vi "write memory.vi"(8 "error in (no error)":errorcluster, 10 "IQ data":u64[](array[numeric]), 11 "USRP_1_x_200MHz in":refnum<class "USRP_1_x_200MHz.lvclass">) -> (0 "error out":errorcluster, 3 "USRP_1_x_200MHz out":refnum<class "USRP_1_x_200MHz.lvclass">)   [LabVIEW 2021, in "USRP_1_x_200MHz.lvclass"]
uses:
  USRP_1_x_200MHz.lvclass
  USRP_1_x_200MHz.lvclass/USRP_1_x_200MHz.ctl
  <vilib>/rvi/interface/nirviMethod/nirviMethod.xnode
  <vilib>/FPGAPlugInAG/Dynamic/niLvFpga_WriteFifo_Dynamic.vi
  <vilib>/rvi/errors/niLvFpgaMergeErrorWithErrorCode.vi
  <vilib>/FPGAPlugInAG/Dynamic/niLvFpga_ConfigureFifo_Dynamic.vi
  <vilib>/FPGAPlugInAG/Dynamic/niLvFpga_StopFifo_Dynamic.vi
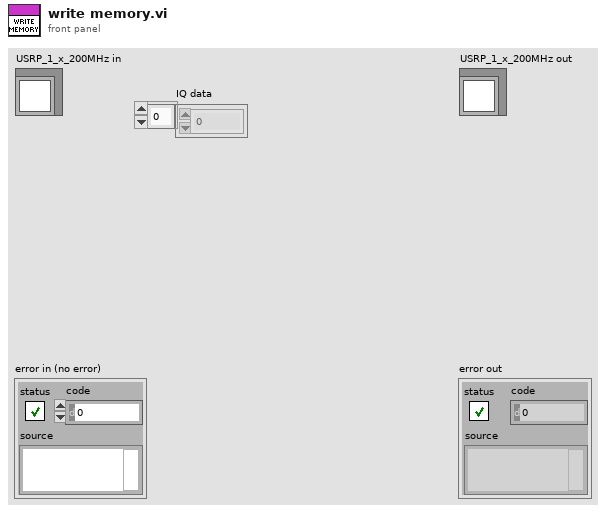
[diagram p1: front panel]
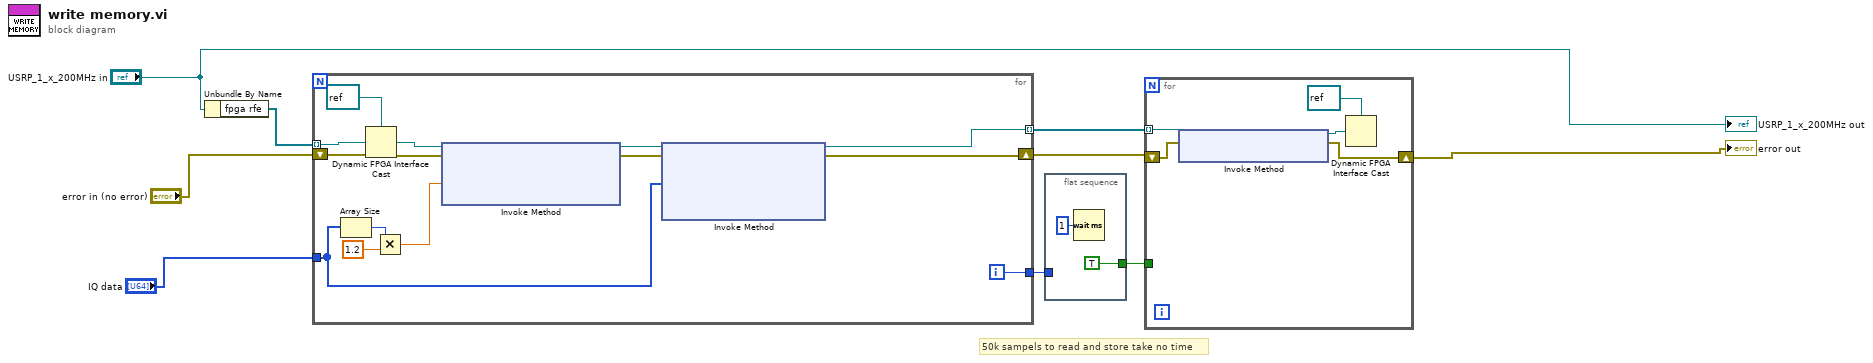
[diagram p0: block diagram]
diagram:
  # "50k sampels to read and store take no time"
  n1 = Unbundle By Name("USRP_1_x_200MHz in") -> ("fpga rfe"=w9:refnum<k20>[])
  n2 = for {
    tunnel: w9 -> [w12] mode=indexing
    shift-right: [w21] -> w7
    shift-left: "error in (no error)" -> [w17]
    tunnel: [w22] -> w8 mode=indexing
    tunnel: [w14] -> w5
    tunnel: "IQ data" -> [w13]
    i -> [w14]
    n3 = Array Size(array=w13) -> (size(s)=w20:i32)
    n4 = Dynamic FPGA Interface Cast(Session In=refnum<k20> refnum ("Type"), Type=w12) -> (Session Out=w11:refnum<k20>)
    n5 = Multiply(x=w20, y=1.2) -> (x*y=w19:dbl)
    n6 = xnode "Invoke Method"("FPGA VI Reference In"=w11, "error in"=w17, "Requested Depth"=w19) -> ("FPGA VI Reference Out"=w16:refnum<k20>, "error out"=w15:errorcluster)  [unwired: 1 out]
    n7 = xnode "Invoke Method"("FPGA VI Reference In"=w16, "error in"=w15, "Data"=w13) -> ("FPGA VI Reference Out"=w22:refnum<k20>, "error out"=w21:errorcluster)  [unwired: 1 in, 1 out]
  }
  n8 = flat-sequence {
    tunnel: [TRUE] -> w6
    tunnel: w5 -> [_]
    frame #0 {
      n9 = Wait (ms)(milliseconds to wait=u32 1) -> ()  [unwired: 1 out]
    }
  }
  n10 = for {
    tunnel: w8 -> [w29] mode=indexing
    shift-right: [w27] -> w4
    shift-left: w7 -> [w28]
    tunnel: w6 -> [_]
    n11 = xnode "Invoke Method"("FPGA VI Reference In"=w29, "error in"=w28) -> ("FPGA VI Reference Out"=w26:refnum<k20>, "error out"=w27:errorcluster)
    n12 = Dynamic FPGA Interface Cast(Session In=refnum<k20> refnum ("FPGA VI Reference Out"), Type=w26) -> ()  [unwired: 1 out]
  }
  "error out" <- w4
  "USRP_1_x_200MHz out" <- "USRP_1_x_200MHz in"
